vi "Write conn.vi"(8 "error in (no error)":errorcluster, 10 "conn":u64, 11 "SP in":refnum<class "Save messages PGserver.lvclass">) -> (0 "error out":errorcluster, 3 "SP out":refnum<class "Save messages PGserver.lvclass">)   [LabVIEW 2019, in "Save messages PGserver.lvclass"]
uses:
  Save messages PGserver.lvclass
  Save messages PGserver.lvclass/Save messages PGserver.ctl
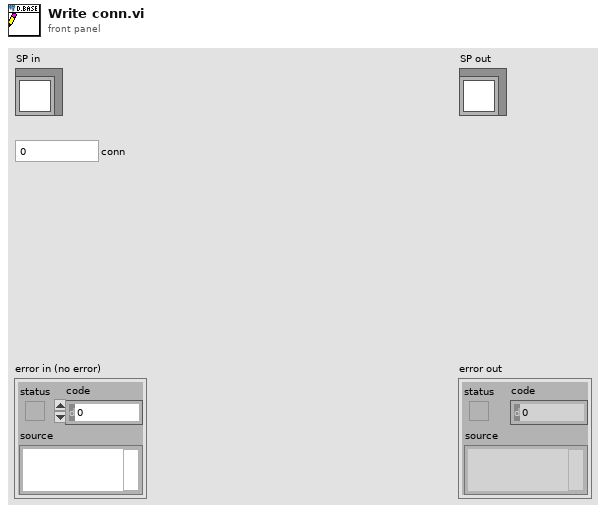
[diagram p1: front panel]
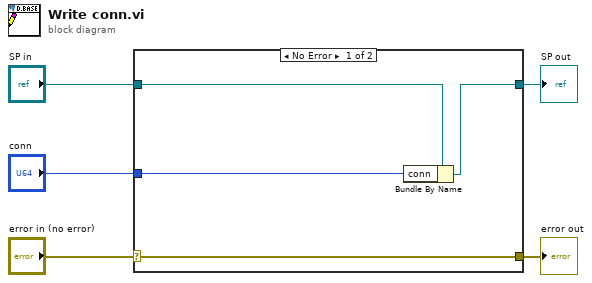
[diagram p0: block diagram]
diagram:
  n1 = case shown="No Error" "error in (no error)" {
    selector: "error in (no error)" -> [w9 w10]
    tunnel: [w9 w10] -> w4
    tunnel: [w7 w11] -> w2
    tunnel: "SP in" -> [w8 w11]
    tunnel: "conn" -> [w6 _]
    frame No Error {
      n2 = Bundle By Name(cluster=w8, "conn"=w6) -> (w7:refnum<class "Save messages PGserver.lvclass">)
    }
    frame Error {
    }
  }
  "error out" <- w4
  "SP out" <- w2
